vi "DSF.Engine.Plugin.Initialize.vi"(8 "error in (no error)":errorcluster, 11 "PXImc Plugin in":refnum<class "DSF.Plugin.PXImc.lvclass">) -> (0 "error out":errorcluster, 3 "PXImc Plugin out":refnum<class "DSF.Plugin.PXImc.lvclass">)   [LabVIEW 2017, in "DSF.Plugin.PXImc.lvclass"]
uses:
  DSF.Plugin.PXImc.lvclass
  Engine/Classes/Plugin/Plugin.lvclass
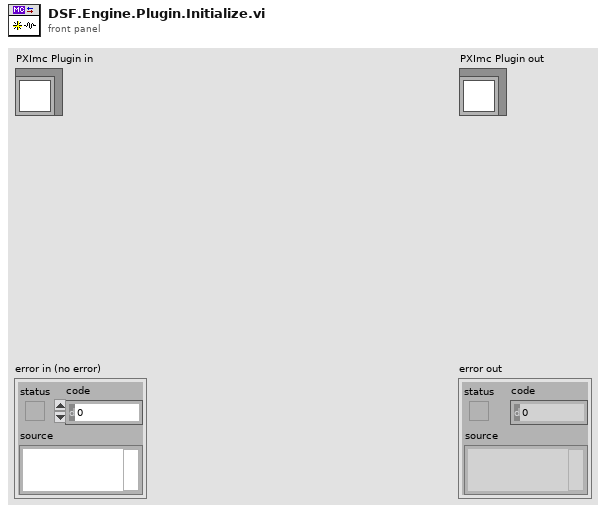
[diagram p1: front panel]
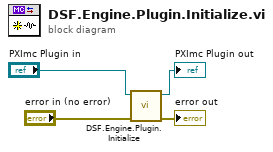
[diagram p0: block diagram]
diagram:
  n1 = call-parent "DSF.Engine.Plugin.Initialize.vi"("error in (no error)"="error in (no error)", "Plugin in"="PXImc Plugin in") -> ("error out"=→"error out":errorcluster, "Plugin out"=→"PXImc Plugin out":refnum<class "DSF.Plugin.PXImc.lvclass">)  [unwired: 8 in]
